vi "Trigger_Camera_Poin_Measurement.vi"(0 "error out 2":errorcluster) -> (2 "error out":errorcluster, 3 "Number Of Pulses":i32, 4 "task out":refnum<k21>)   [LabVIEW 2011]
uses:
  Program Files/National Instruments/LabVIEW 2011/resource/objmgr/daqmx.rc
  Variables/GlobalSetGetTriggerForPointMeasurement.vi
  <vilib>/DAQmx/configure/trigger.llb/DAQmx Start Trigger (Digital Edge).vi
  <vilib>/DAQmx/configure/timing.llb/DAQmx Timing (Implicit).vi
  <vilib>/DAQmx/create/channels.llb/DAQmx Create Channel (CO-Pulse Generation-Frequency).vi
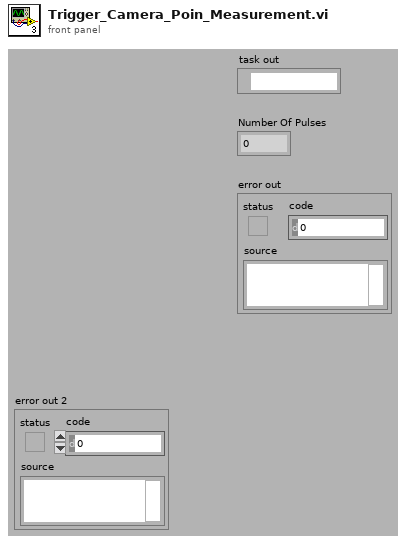
[diagram p1: front panel]
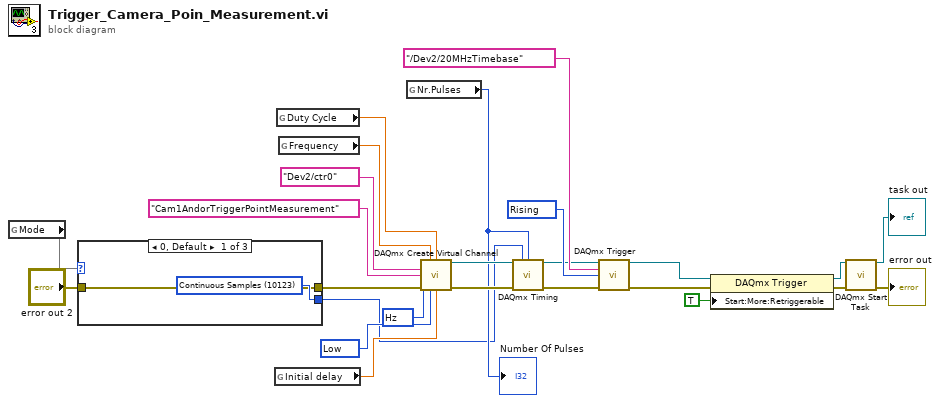
[diagram p0: block diagram]
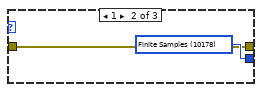
[diagram p2: hidden frame]
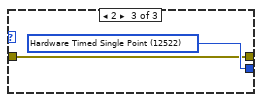
[diagram p3: hidden frame]
diagram:
  w1 = 10373 items=["Hz"=10373] ("units")
  w15 = 10280 items=["Rising"=10280, "Falling"=10171] ("Trigger Edge")
  w12 = 10214 items=["High"=10192, "Low"=10214] ("Idle State")
  n1 = global read "GlobalSetGetTriggerForPointMeasurement.vi" "Mode"() -> (w5)
  n2 = case shown="0, Default" w5 {
    tunnel: [w27 w29 w31] -> w4
    tunnel: [w26 w28 w30] -> w3
    tunnel: "error out 2" -> [w26 w28 w30]
    frame 0, Default {
      w27 = 10123 items=["Finite Samples"=10178, "Continuous Samples"=10123, "Hardware Timed Single Point"=12522] ("Mode")
    }
    frame 1 {
      w29 = 10178 items=["Finite Samples"=10178, "Continuous Samples"=10123, "Hardware Timed Single Point"=12522] ("Mode")
    }
    frame 2 {
      w31 = 12522 items=["Finite Samples"=10178, "Continuous Samples"=10123, "Hardware Timed Single Point"=12522] ("Mode")
    }
  }
  n3 = global read "GlobalSetGetTriggerForPointMeasurement.vi" "Initial delay"() -> (w9:dbl)
  n4 = global read "GlobalSetGetTriggerForPointMeasurement.vi" "Duty Cycle"() -> (w8:dbl)
  n5 = global read "GlobalSetGetTriggerForPointMeasurement.vi" "Frequency"() -> (w6:dbl)
  n6 = global read "GlobalSetGetTriggerForPointMeasurement.vi" "Nr.Pulses"() -> (w7:i32)
  "Number Of Pulses" <- w7
  n7 = call-poly <vilib>:"DAQmx Create Virtual Channel.vi"("frequency"=w6, "duty cycle"=w8, "counter"=tag "Dev2/ctr0", "name to assign"="Cam1AndorTriggerPointMeasurement", "units"=w1, "error in"=w3, "idle state"=w12, "initial delay"=w9) -> ("task out"=w11:refnum<k21>, "error out"=w10:errorcluster)  [unwired: 6 in]
  n8 = call-poly <vilib>:"DAQmx Timing.vi"("task/channels in"=w11, "sample mode"=w4, "samples per channel"=w7, "error in"=w10) -> ("task out"=w13:refnum<k21>, "error out"=w14:errorcluster)  [unwired: 10 in]
  n9 = call-poly <vilib>:"DAQmx Trigger.vi"("task/channels in"=w13, "source"=tag "/Dev2/20MHzTimebase", "edge"=w15, "error in"=w14) -> ("task out"=w17:refnum<k21>, "error out"=w18:errorcluster)  [unwired: 10 in]
  n10 = property class="DAQmx Trigger"(reference=w17, error in=w18, "Start:More:Retriggerable"=TRUE) -> (reference out=w20:refnum<k21>, error out=w25:errorcluster)
  n11 = call <vilib>:"DAQmx Start Task.vi"("task/channels in"=w20, "error in"=w25) -> ("task out"=→"task out":refnum<k21>, "error out"=→"error out":errorcluster)  [unwired: 12 in]
